vi "Generate Test Data.vi"(11 "M data in":refnum<class "M data.lvclass">) -> (3 "M data out":refnum<class "M data.lvclass">)   [LabVIEW 2014, in "Alicat Lib.lvlib" / "M data.lvclass"]
uses:
  M data.lvclass
  M data.lvclass/M data.ctl
  Alicat Data.lvclass
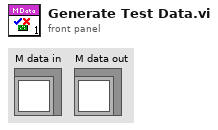
[diagram p1: front panel]
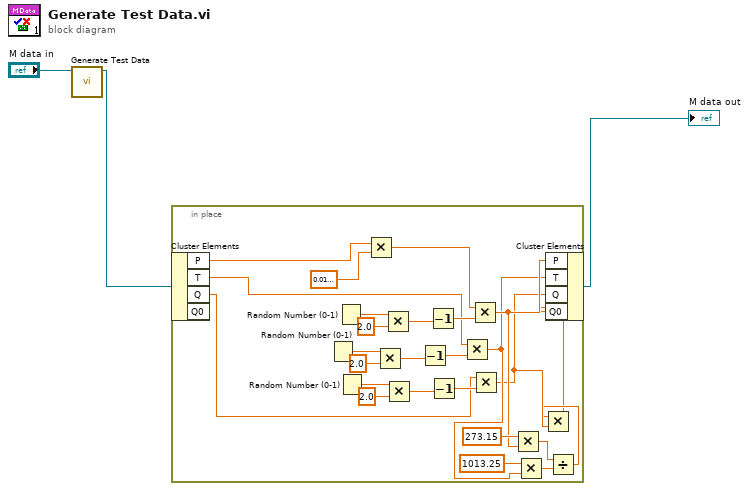
[diagram p0: block diagram]
diagram:
  n1 = call-parent "Generate Test Data.vi"("Alicat Data in"="M data in") -> ("Alicat Data out"=w2:refnum<class "M data.lvclass">)  [unwired: 10 in]
  n2 = in-place {
    n3 = in-place-cluster #1(w2) -> ("P"=w23:sgl, "T"=w14:sgl, "Q"=w13:sgl)  [unwired: 1 out]
    n4 = Random Number (0-1)() -> (number: 0 to 1=w15:dbl)
    n5 = Random Number (0-1)() -> (number: 0 to 1=w28:dbl)
    n6 = Random Number (0-1)() -> (number: 0 to 1=w19:dbl)
    n7 = Multiply(x=w23, y=sgl 0.02) -> (x*y=w24:sgl)
    n8 = Multiply(x=w15, y=2.0) -> (x*y=w17:dbl)
    n9 = Multiply(x=w28, y=2.0) -> (x*y=w26:dbl)
    n10 = Multiply(x=w19, y=2.0) -> (x*y=w21:dbl)
    n11 = Decrement(x=w17) -> (x-1=w18:dbl)
    n12 = Decrement(x=w26) -> (x-1=w25:dbl)
    n13 = Decrement(x=w21) -> (x-1=w22:dbl)
    n14 = Multiply(x=w14, y=w18) -> (x*y=w8:dbl)
    n15 = Multiply(x=w24, y=w25) -> (x*y=w11:dbl)
    n16 = Multiply(x=w13, y=w22) -> (x*y=w6:dbl)
    n17 = Multiply(x=273.15, y=w11) -> (x*y=w10:dbl)
    n18 = Multiply(x=1013.25, y=w8) -> (x*y=w7:dbl)
    n19 = Divide(x=w10, y=w7) -> (x/y=w5:dbl)
    n20 = Multiply(x=w5, y=w6) -> (x*y=w4:dbl)
    n21 = in-place-cluster #1("P"=w11, "T"=w8, "Q"=w6, "Q0"=w4) -> (→"M data out":refnum<class "M data.lvclass">)
  }
